vi "p1.vi"() -> ()   [LabVIEW 2023, in "d14.lvlib"]
uses:
  d14.lvlib
  AOC/AOC.lvlib
panel:
  out "Answer":u64
  in  "Example":string="O....#....\nO.OO#....#\n.....##...\nOO.#O....O\n.O.....O#.\nO.#..O.#.#\n..O..#O..O\n.......O..\n#....###..\n#OO..#...."
  in  "Example":bool
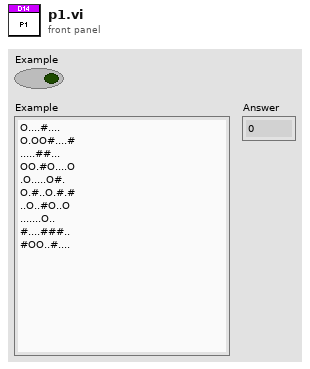
[diagram p1: front panel]
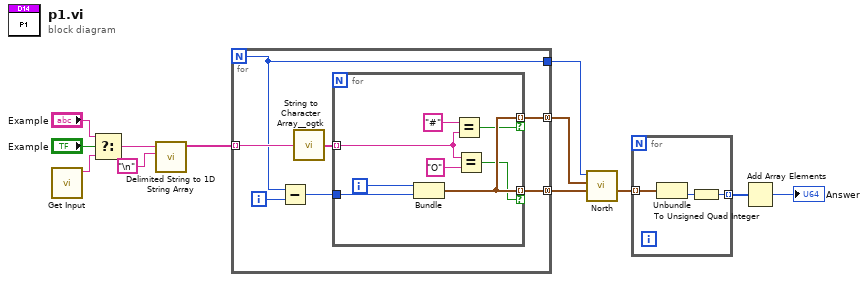
[diagram p0: block diagram]
diagram:
  n1 = call "Get Input.vi"() -> ("Input"=w12:string)  [unwired: 11 in]
  n2 = Select(t="Example", s="Example", f=w12) -> (s? t:f=w9:string)
  n3 = call <vilib>:"Delimited String to 1D String Array.vi"("delimiter"="\n", "delimited string"=w9) -> ("string array"=w7:string[])  [unwired: 9 in]
  n4 = for {
    N -> [w13]
    tunnel: w7 -> [w19] mode=indexing
    tunnel: [w17] -> w6 mode=concatenating
    tunnel: [w16] -> w5 mode=concatenating
    tunnel: [w13] -> w4
    i -> [w15]
    n5 = Subtract(x=w13, y=w15) -> (x-y=w14:i32)
    n6 = call <userlib>:"String to Character Array__ogtk.vi"("Input String"=w19) -> ("Character Array"=w18:string[])
    n7 = for {
      tunnel: w18 -> [w22] mode=indexing
      tunnel: w14 -> [w26]
      tunnel: [w25] -> w16 mode=indexing if=w20
      tunnel: [w25] -> w17 mode=indexing if=w23
      i -> [w27]
      n8 = Bundle(w27, w26) -> (w25:cluster{i32, i32})  [unwired: 1 in]
      n9 = Equal?(x="#", y=w22) -> (x = y?=w23:bool)
      n10 = Equal?(x=w22, y="O") -> (x = y?=w20:bool)
    }
  }
  n11 = call "North.vi"("Spheres in"=w5, "Cubes"=w6, "Northmost"=w4) -> ("Spheres out"=w1:cluster{i32, i32}[])  [unwired: 8 in]
  n12 = for {
    tunnel: w1 -> [w30] mode=indexing
    tunnel: [w28] -> w3 mode=indexing
    n13 = Unbundle(w30) -> (w29:i32)  [unwired: 1 out]
    n14 = To Unsigned Quad Integer(1:w29) -> (0:w28:u64)
  }
  n15 = Add Array Elements(numeric array=w3) -> (sum=→"Answer":u64)
